vi "Benchmark inline subVI call.vi"() -> ()   [LabVIEW 2016]
panel:
  out "us/iteration":dbl format="%.6f"
  in  "iterations":i32=1000000000
  # "0.001259 us/iteration 1E9 iterations"
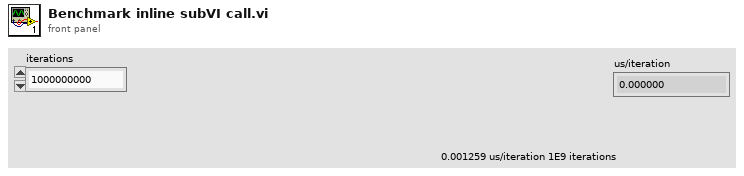
[diagram p1: front panel]
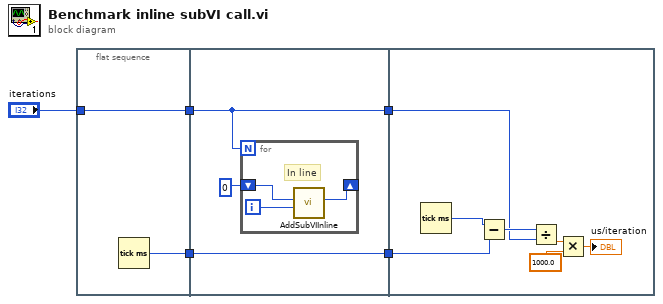
[diagram p0: block diagram]
diagram:
  n1 = flat-sequence {
    tunnel: [w7] -> w5
    tunnel: [w6] -> w2
    tunnel: "iterations" -> [w6]
    tunnel: w5 -> [w10]
    tunnel: [w10] -> w4
    tunnel: [w8] -> w3
    tunnel: w2 -> [w8]
    tunnel: w4 -> [w19]
    tunnel: w3 -> [w17]
    frame #0 {
      n2 = Tick Count (ms)() -> (millisecond timer value=w7:u32)
    }
    frame #1 {
      n3 = for {
        N: w8 -> [_]
        shift-right: [w11] -> _
        shift-left: 0 -> [w12]
        i -> [w13]
        # "In line"
        n4 = call "AddSubVIInline.vi"("Numeric 3"=w13, "Numeric in"=w12) -> ("Numeric out"=w11:i32)  [unwired: 9 in]
      }
    }
    frame #2 {
      n5 = Tick Count (ms)() -> (millisecond timer value=w20:u32)
      n6 = Subtract(x=w20, y=w19) -> (x-y=w18:u32)
      n7 = Divide(x=w18, y=w17) -> (x/y=w16:dbl)
      n8 = Multiply(x=w16, y=1000.0) -> (x*y=→"us/iteration":dbl)
    }
  }
